vi "calibrateJuicer.vi"(6 "Time Stamp":timestamp, 7 "Window Number (0...15)":i32, 8 "error in (no error)":errorcluster, 9 "ISI":dbl, 10 "Pulse duration":dbl, 11 "Juicer in":refnum<class "Juicer.lvclass">) -> (0 "error out":errorcluster, 1 "Time Stamp 2":timestamp, 3 "Juicer out":refnum<class "Juicer.lvclass">)   [LabVIEW 2014, in "Juicer.lvclass"]
uses:
  Juicer.lvclass
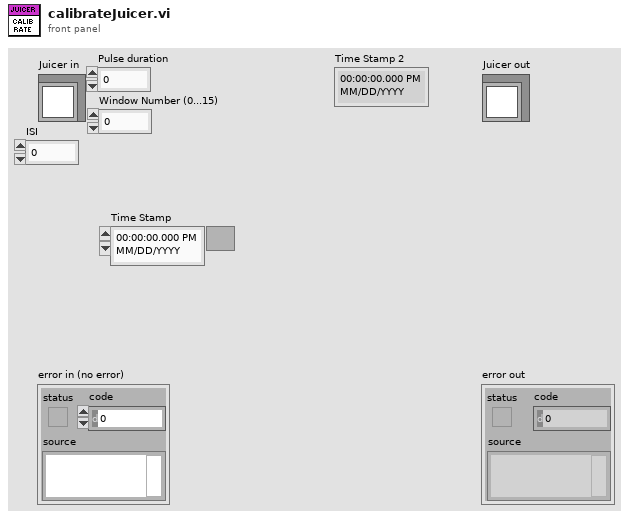
[diagram p1: front panel]
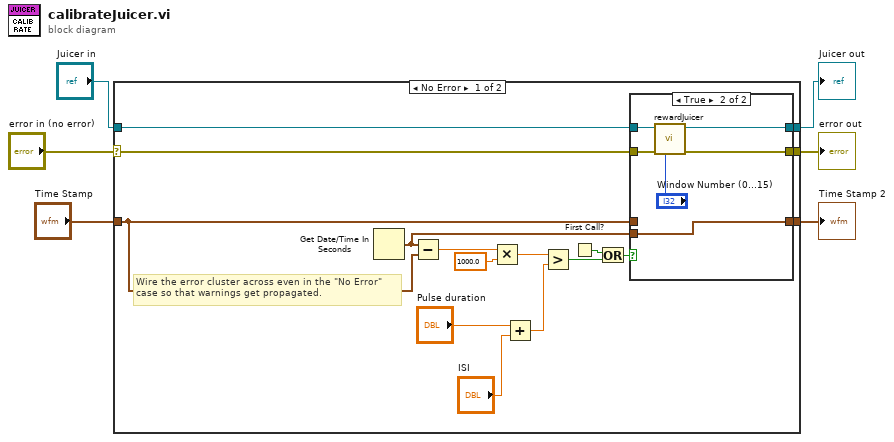
[diagram p0: block diagram]
diagram:
  n1 = case shown="No Error" "error in (no error)" {
    selector: "error in (no error)" -> [w20 w34]
    tunnel: [w19 w34] -> w5
    tunnel: [w21 w33] -> w3
    tunnel: "Juicer in" -> [w22 w33]
    tunnel: "Time Stamp" -> [w10 w32]
    tunnel: [w12 w32] -> w1
    frame No Error {
      # "Wire the error cluster across even in the \"No Error\"\ncase so that warnings get propagated."
      n2 = Get Date/Time In Seconds() -> (seconds since 1Jan1904=w11:timestamp)
      n3 = Subtract(x=w11, y=w10) -> (x-y=w9:dbl)
      n4 = Multiply(x=w9, y=1000.0) -> (x*y=w8:dbl)
      n5 = Add(x="Pulse duration", y="ISI") -> (x+y=w18:dbl)
      n6 = Greater?(x=w8, y=w18) -> (0:w16:bool)
      n7 = First Call?() -> (First Call?: T/F=w15:bool)
      n8 = Or(x=w15, y=w16) -> (x .or. y?=w17:bool)
      n9 = case shown="True" w17 {
        tunnel: w22 -> [w25 w31]
        tunnel: [w25 w30] -> w21
        tunnel: w20 -> [w24 w29]
        tunnel: [w24 w28] -> w19
        tunnel: w10 -> [w23 _]
        tunnel: [w23 w27] -> w12
        tunnel: w11 -> [_ w27]
        frame False {
        }
        frame True {
          n10 = call-dynamic "rewardJuicer.vi"("error in (no error)"=w29, "Window Number (0...15)"="Window Number (0...15)", "Juicer in"=w31) -> ("error out"=w28:errorcluster, "Juicer out"=w30:refnum<class "Juicer.lvclass">)  [unwired: 6 in, 1 out]
        }
      }
    }
    frame Error {
    }
  }
  "error out" <- w5
  "Juicer out" <- w3
  "Time Stamp 2" <- w1
